vi "check_for_image_pixel.vi"(10 "i32_ar_first_and_last_pixel":i32[](array[numeric]), 11 "current index":i32) -> (3 "image pixel":bool)   [LabVIEW 2011]
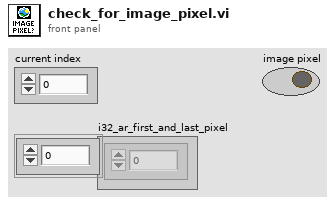
[diagram p1: front panel]
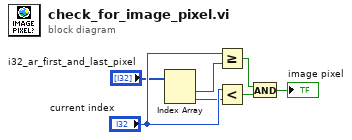
[diagram p0: block diagram]
diagram:
  n1 = Index Array(array="i32_ar_first_and_last_pixel") -> (element #1=w2:i32, element #2=w1:i32)  [unwired: 2 in]
  n2 = Greater Or Equal?(x="current index", y=w2) -> (x >= y?=w3:bool)
  n3 = Less?(x="current index", y=w1) -> (x < y?=w4:bool)
  n4 = And(x=w3, y=w4) -> (x .and. y?=→"image pixel":bool)
